vi "Write File.vi"(8 "error in (no error)":errorcluster, 10 "path":path, 11 "xwpfWriter in":refnum<class "xwpfWriter.lvclass">) -> (0 "error out":errorcluster, 3 "xwpfWriter out":refnum<class "xwpfWriter.lvclass">)   [LabVIEW 2017, in "xwpfWriter.lvclass"]
uses:
  xwpfWriter.lvclass
  xwpfWriter.lvclass/xwpfWriter.ctl
  C:/Users/Neo/Desktop/Dev_Tools_BR/LabVIEW_NPOI/lib/NPOI 2.1.1/NPOI.OOXML.dll
  lib/NPOI 2.1.1/NPOI.OOXML.dll
  Support/File Stream/File Stream.lvlib
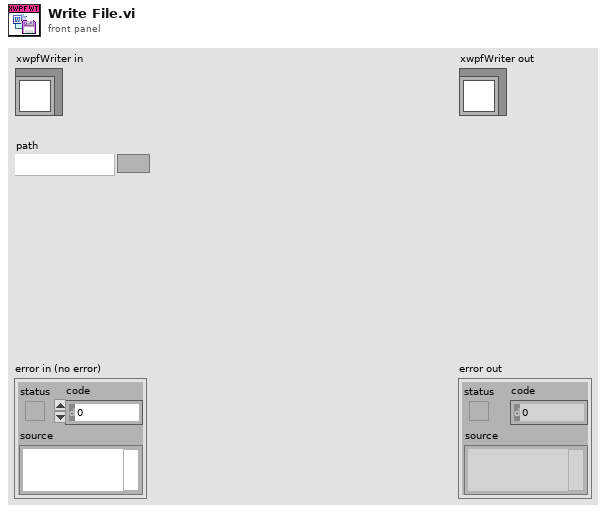
[diagram p1: front panel]
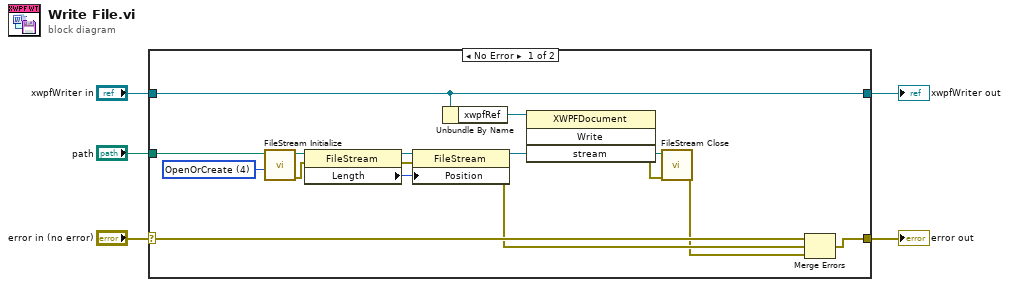
[diagram p0: block diagram]
diagram:
  n1 = case shown="No Error" "error in (no error)" {
    selector: "error in (no error)" -> [w20 w22]
    tunnel: [w17 w22] -> w4
    tunnel: [w19 w21] -> w2
    tunnel: "xwpfWriter in" -> [w19 w21]
    tunnel: "path" -> [w14 _]
    frame No Error {
      w11 = 4 items=["CreateNew"=1, "Create"=2, "Open"=3, "OpenOrCreate"=4, "Truncate"=5, "Append"=6] ("mode")
      n2 = call "FileStream Initialize.vi"("mode"=w11, "path"=w14) -> ("error out"=w9:errorcluster, "new reference"=w13:refnum<k24>)  [unwired: 8 in]
      n3 = property class="FileStream"(reference=w13, error in=w9) -> (reference out=w16:refnum<k24>, error out=w10:errorcluster, "Length"=w15:i64)
      n4 = property class="FileStream"(reference=w16, error in=w10, "Position"=w15) -> (reference out=w12:refnum<k24>, error out=w7:errorcluster)
      n5 = Unbundle By Name(w19) -> ("xwpfRef"=w18:refnum<k24>)
      n6 = invoke class="XWPFDocument" method="Write"(reference=w18, "stream"=w12) -> (error out=w8:errorcluster)  [unwired: 2 in, 3 out]
      n7 = call "FileStream Close.vi"("error in (no error)"=w8, "reference"=w12) -> ("error out"=w6:errorcluster)  [unwired: 9 in]
      n8 = Merge Errors(w20, w7, w6) -> (w17:errorcluster)
    }
    frame Error {
    }
  }
  "error out" <- w4
  "xwpfWriter out" <- w2
